vi "Check if Dashboard is connected to the robot (Dashboard).vi"(8 "From shift":dbl) -> (0 "to shift":dbl, 3 "Number Changing":bool)   [LabVIEW 2013]
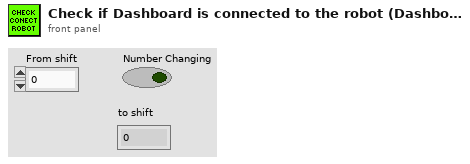
[diagram p1: front panel]
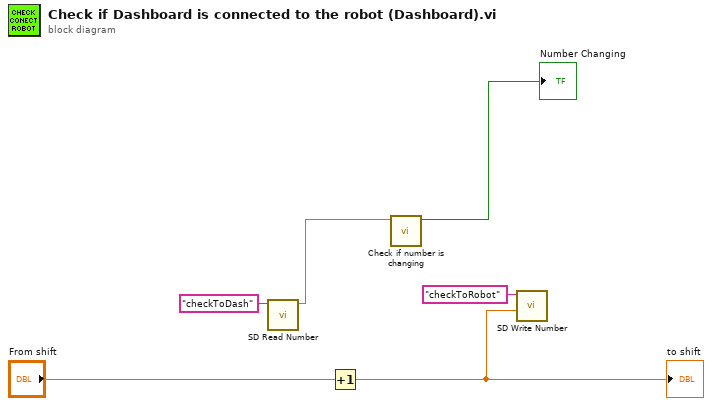
[diagram p0: block diagram]
diagram:
  n1 = call <vilib>:"SD Read Number.vi"("Name"="checkToDash") -> ("Numeric"=w2:dbl)  [unwired: 8 in, 2 out]
  n2 = Increment(x="From shift") -> (x+1=w5:dbl)
  "to shift" <- w5
  n3 = call "Check if number is changing.vi"("Number to check"=w2) -> ("Number Changing"=→"Number Changing":bool)  [unwired: 9 in, 1 out]
  n4 = call <vilib>:"SD Write Number.vi"("Numeric"=w5, "Name"="checkToRobot") -> ()  [unwired: 8 in, 2 out]
